vi "FindMostRecentFile.vi"() -> ()   [LabVIEW 2018]
uses:
  406562c1-697f-4648-b42d-40e5e1d0334e.vi
  <vilib>/Array/Sort 2D Array - Pop Stack.vi
  <vilib>/Array/Sort 2D Array - Push Stack.vi
panel:
  in  "line index":i32(ring) items=["INPUT", "OUTPUT"]
  out "Newest File":string
  out "sorted 2D array":string[][](array[string])
  out "Array":string[](array[string])
  out "Time(num)":dbl[](array[numeric])
  out "Timestamp":timestamp[](array[timestamp])
  out "Filtered Files":string[](array[string])
  out "array":string[](array[string])
  out "standard output":string
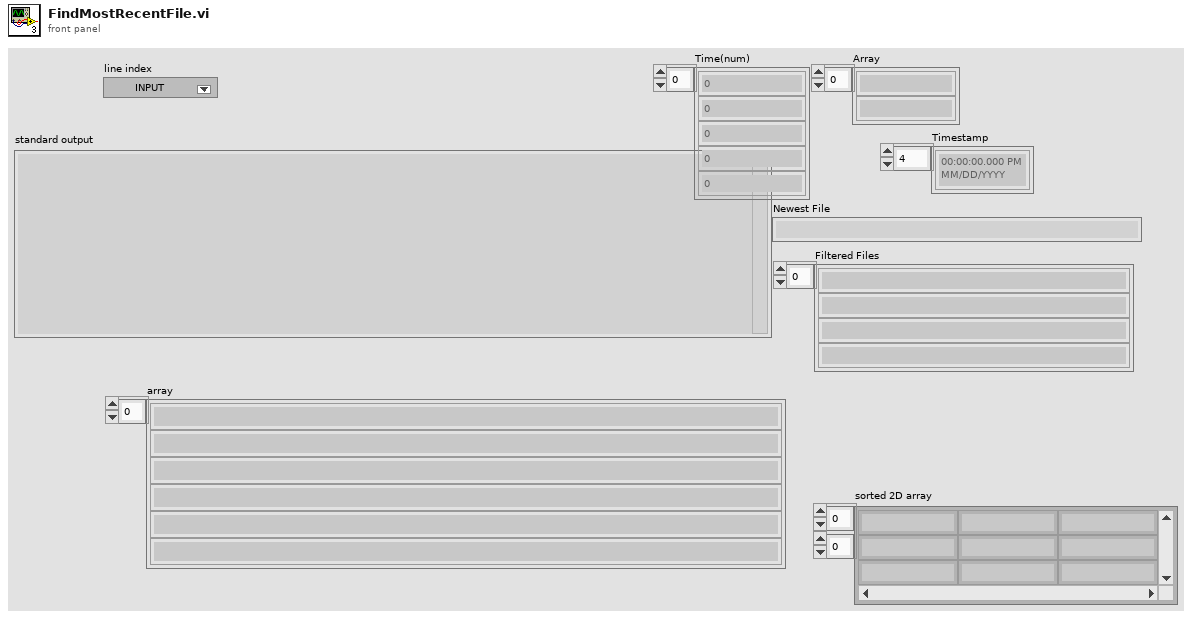
[diagram p1: front panel]
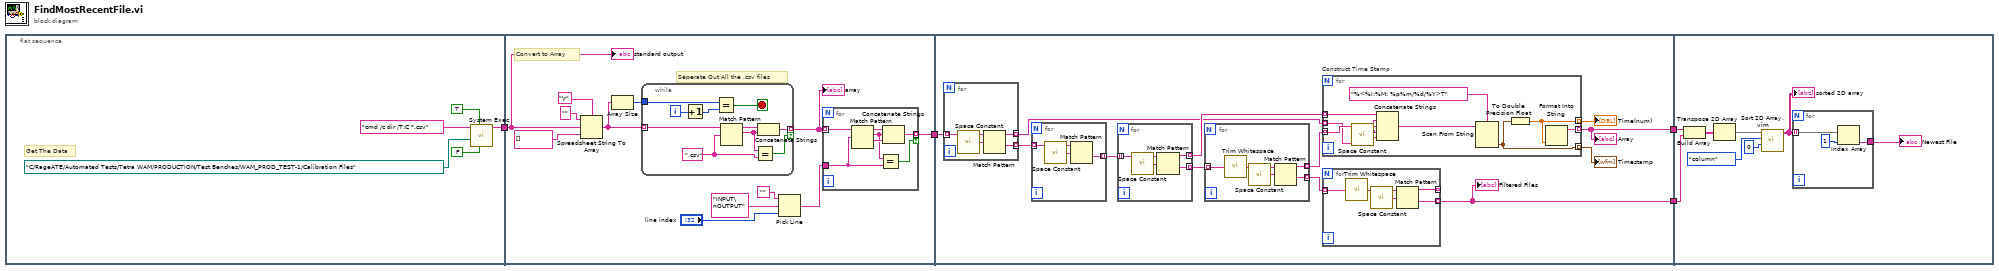
[diagram p0: block diagram]
diagram:
  n1 = flat-sequence {
    tunnel: [w5] -> w4
    tunnel: w4 -> [w19]
    tunnel: [w14] -> w3
    tunnel: w3 -> [w50]
    tunnel: [w41] -> w2
    tunnel: [w39] -> w1
    tunnel: w2 -> [w87]
    tunnel: w1 -> [w88]
    frame #0 {
      # "Get The Data"
      n2 = call <vilib>:"System Exec.vi"("run minimized? (F)"=FALSE, "wait until completion? (T)"=TRUE, "working directory"=path "C:/RageATE/Automated Tests/Tetra WAM/PRODUCTION/Test Benches/WAM_PROD_TEST-1/Calibration Files", "command line"="cmd /c dir /T:C *.csv") -> ("standard output"=w5:string)  [unwired: 4 in, 3 out]
    }
    frame #1 {
      # "Convert to Array"
      # "Seperate Out All the .csv files"
      n3 = Spreadsheet String To Array(delimiter (Tab)="\r", format string="", spreadsheet string=w19, array type (2D Dbl)=string[] []) -> (array=w17:string[])
      n4 = Array Size(array=w17) -> (size(s)=w16:i32)
      n5 = while {
        tunnel: w17 -> [w38] mode=indexing
        tunnel: [w36] -> w15 mode=indexing if=w35
        tunnel: w16 -> [w31]
        i -> [w30]
        stop <- w32 stop-if-true
        w33 = ".csv" ("regular expression")
        n6 = Increment(x=w30) -> (x+1=w29:i32)
        n7 = Equal?(x=w31, y=w29) -> (x = y?=w32:bool)
        n8 = Match Pattern(string=w38, regular expression=w33) -> (before substring=w37:string, match substring=w34:string)  [unwired: 1 in, 2 out]
        n9 = Equal?(x=w34, y=w33) -> (x = y?=w35:bool)
        n10 = Concatenate Strings(w37, w34) -> (w36:string)
      }
      "array" <- w15
      n11 = Pick Line(string ("")="", multi-line string="INPUT\nOUTPUT", line index="line index") -> (output string=w11:string)
      n12 = for {
        tunnel: w15 -> [w28] mode=indexing
        tunnel: w11 -> [w24]
        tunnel: [w23] -> w14 mode=indexing if=w22
        n13 = Match Pattern(string=w28, regular expression=w24) -> (before substring=w27:string, match substring=w25:string, after substring=w26:string)  [unwired: 1 in, 1 out]
        n14 = Equal?(x=w25, y=w24) -> (x = y?=w22:bool)
        n15 = Concatenate Strings(w27, w25, w26) -> (w23:string)
      }
      "standard output" <- w19
    }
    frame #2 {
      n16 = for {
        tunnel: w50 -> [w80] mode=indexing
        tunnel: [w78] -> w44 mode=indexing
        tunnel: [w77] -> w49 mode=indexing
        n17 = call <vilib>:"Space Constant.vi"() -> ("String"=w79:string)
        n18 = Match Pattern(string=w80, regular expression=w79) -> (before substring=w78:string, after substring=w77:string)  [unwired: 1 in, 2 out]
      }
      n19 = for {
        tunnel: w49 -> [w76] mode=indexing
        tunnel: [w74] -> w48 mode=indexing
        n20 = call <vilib>:"Space Constant.vi"() -> ("String"=w75:string)
        n21 = Match Pattern(string=w76, regular expression=w75) -> (after substring=w74:string)  [unwired: 1 in, 3 out]
      }
      n22 = for {
        tunnel: w48 -> [w73] mode=indexing
        tunnel: [w71] -> w45 mode=indexing
        tunnel: [w70] -> w47 mode=indexing
        n23 = call <vilib>:"Space Constant.vi"() -> ("String"=w72:string)
        n24 = Match Pattern(string=w73, regular expression=w72) -> (before substring=w71:string, after substring=w70:string)  [unwired: 1 in, 2 out]
      }
      n25 = for {
        tunnel: w47 -> [w69] mode=indexing
        tunnel: [w67] -> w43 mode=indexing
        tunnel: [w66] -> w46 mode=indexing
        n26 = call <vilib>:"Trim Whitespace.vi"("string"=w69) -> ("trimmed string"=w65:string)  [unwired: 1 in]
        n27 = call <vilib>:"Space Constant.vi"() -> ("String"=w68:string)
        n28 = Match Pattern(string=w65, regular expression=w68) -> (before substring=w67:string, after substring=w66:string)  [unwired: 1 in, 2 out]
      }
      n29 = for "Construct Time Stamp" {
        tunnel: w45 -> [w57] mode=indexing
        tunnel: w44 -> [w54] mode=indexing
        tunnel: [w53] -> w42 mode=indexing
        tunnel: w43 -> [w56] mode=indexing
        tunnel: [w52] -> w40 mode=indexing
        tunnel: [w51] -> w39 mode=indexing
        n30 = call <vilib>:"Space Constant.vi"() -> ("String"=w55:string)
        n31 = Concatenate Strings(w57, w55, w56, w55, w54) -> (w59:string)
        n32 = Scan From String(format string="%<%I:%M: %p%m/%d/%Y>T", input string=w59) -> (output 1=w53:timestamp)  [unwired: 3 in, 3 out]
        n33 = To Double Precision Float(number=w53) -> (double precision float=w52:dbl)
        n34 = Format Into String(w52) -> (resulting string=w51:string)  [unwired: 3 in, 1 out]
      }
      "Timestamp" <- w42
      "Time(num)" <- w40
      "Array" <- w39
      n35 = for {
        tunnel: w46 -> [w64] mode=indexing
        tunnel: [w62] -> _ mode=indexing
        tunnel: [w61] -> w41 mode=indexing
        n36 = call <vilib>:"Trim Whitespace.vi"("string"=w64) -> ("trimmed string"=w60:string)  [unwired: 1 in]
        n37 = call <vilib>:"Space Constant.vi"() -> ("String"=w63:string)
        n38 = Match Pattern(string=w60, regular expression=w63) -> (before substring=w62:string, after substring=w61:string)  [unwired: 1 in, 2 out]
      }
      "Filtered Files" <- w41
    }
    frame #3 {
      n39 = Build Array(w88, w87) -> (w86:string[][])
      n40 = Transpose 2D Array(2D array=w86) -> (transposed array=w85:string[][])
      n41 = call "Sort 2D Array.vim"("index"=0, "dimension to index (column)"=enum16{"column", "row"}."column", "2D array"=w85) -> ("sorted 2D array"=w82:string[][])  [unwired: 7 in, 1 out]
      "sorted 2D array" <- w82
      n42 = for {
        tunnel: w82 -> [w91] mode=indexing
        tunnel: [w89] -> w81
        n43 = Index Array(array=w91, index=1) -> (element=w89:string)
      }
      "Newest File" <- w81
    }
  }
